vi "Fetch.vi"(8 "error in (no error)":errorcluster, 9 "Time Out ( 1000 )":u32=1000, 10 "Fetch Type (0:VOLT)":u16(ring) items=["Voltage", "Max Voltage", "Min Voltage", "Current", "Max Current", "Min Current", "Powers", "Capacity", "Time", "Temperature"], 11 "VISA resource name":refnum<visa-resource-name>) -> (0 "error out":errorcluster, 2 "Data":dbl, 3 "VISA resource name out":refnum<visa-resource-name>)   [LabVIEW 2015, in "IT8900A-E.lvlib"]
doc: "The signal measurement command is used to obtain a reading.You can use this command to control the measurement process.\n\n<b>Fetch Type</b>\n0:Voltage This command is used to read the input voltage of the instrument.\n1:Max Volt This command is used to read the maximum input voltage of the instrument.\n2:Min Volt This command is used to read the minimum input voltage of the instrument. \n3:Current This command is used to read the input current of the instrument.\n4:Max Curr This command is used to read the maximum input current of the instrument.\n5:Min Curr This command is used to read the minimum input current of the instrument.\n6:Power This command is used to read the input power of the instrument.\n7:Capacity This command is used to read the charge and discharge battery capacity. \n8:Time This command is used to read the integral time of the instrument.\n9:Temperature This command is used to obtain cabinet temperature.\n\nDefault : 0:Voltage"
uses:
  <instrlib>/IT8900/IT8900A-E.lvlib
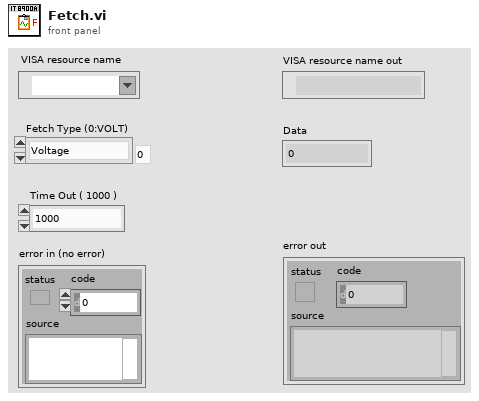
[diagram p1: front panel]
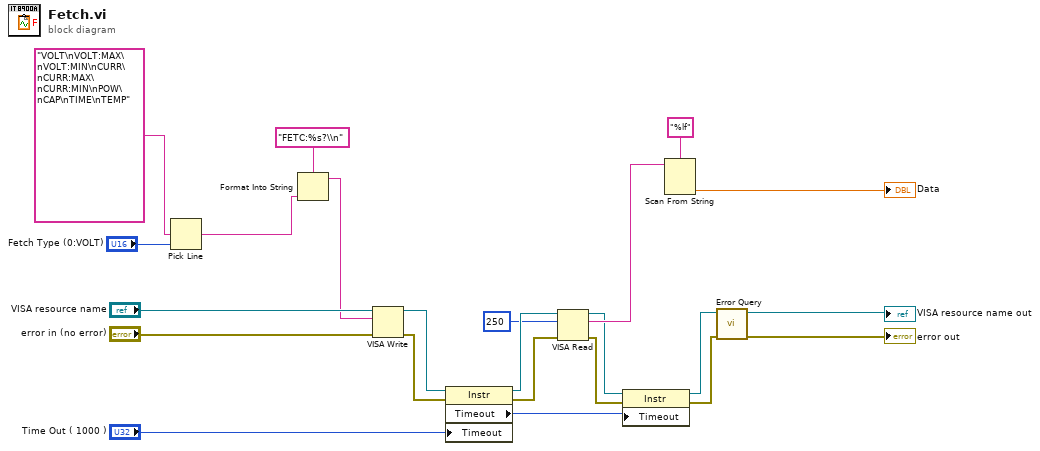
[diagram p0: block diagram]
diagram:
  n1 = Pick Line(multi-line string="VOLT\nVOLT:MAX\nVOLT:MIN\nCURR\nCURR:MAX\nCURR:MIN\nPOW\nCAP\nTIME\nTEMP", line index="Fetch Type (0:VOLT)") -> (output string=w3:string)  [unwired: 1 in]
  n2 = Format Into String(format string="FETC:%s?\\n", w3) -> (resulting string=w22:string)  [unwired: 2 in, 1 out]
  n3 = VISA Write(VISA resource name="VISA resource name", write buffer=w22, error in (no error)="error in (no error)") -> (VISA resource name out=w15:refnum<visa-resource-name>, error out=w13:errorcluster)  [unwired: 1 out]
  n4 = property class="Instr"(reference=w15, error in=w13, "Timeout"="Time Out ( 1000 )") -> (reference out=w14:refnum<visa-resource-name>, error out=w12:errorcluster, "Timeout"=w6:u32)
  n5 = VISA Read(VISA resource name=w14, byte count=u8 250, error in (no error)=w12) -> (VISA resource name out=w11:refnum<visa-resource-name>, read buffer=w20:string, error out=w10:errorcluster)  [unwired: 1 out]
  n6 = property class="Instr"(reference=w11, error in=w10, "Timeout"=w6) -> (reference out=w9:refnum<visa-resource-name>, error out=w8:errorcluster)
  n7 = Scan From String(format string="%lf", input string=w20) -> (output 1=→"Data":dbl)  [unwired: 3 in, 3 out]
  n8 = call <instrlib>:"Error Query.vi"("error in (no error)"=w8, "VISA resource name"=w9) -> ("error out"=→"error out":errorcluster, "VISA resource name out"=→"VISA resource name out":refnum<visa-resource-name>)  [unwired: 6 in, 2 out]
